vi "Shooter Data.vi"(1 "Wheel Speed":T2, 2 "Arm Angle":T1) -> (0 "Shooter Data":T3)   [LabVIEW 2015]
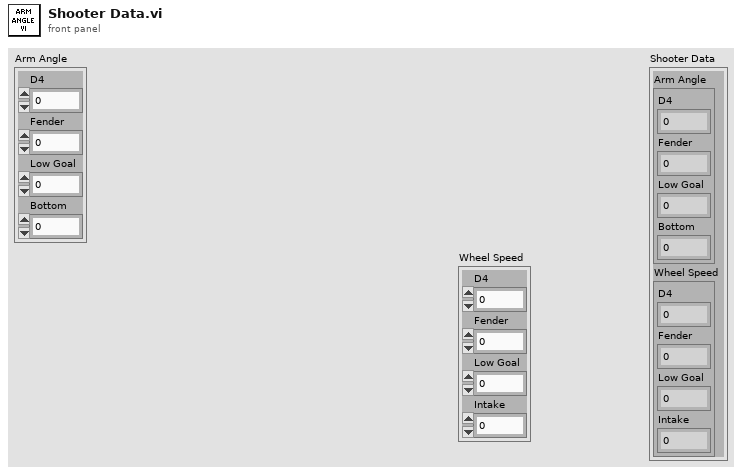
[diagram p1: front panel]
types:
  T1 = cluster{"D4":dbl, "Fender":dbl, "Low Goal":dbl, "Bottom":dbl}
  T2 = cluster{"D4":dbl, "Fender":dbl, "Low Goal":dbl, "Intake":dbl}
  T3 = cluster{"Arm Angle":cluster{"D4":dbl, "Fender":dbl, "Low Goal":dbl, "Bottom":dbl}, "Wheel Speed":cluster{"D4":dbl, "Fender":dbl, "Low Goal":dbl, "Intake":dbl}}
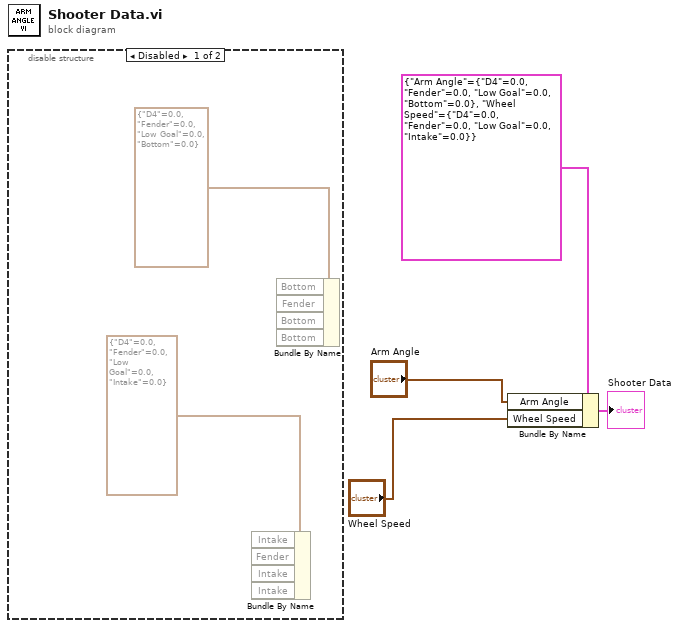
[diagram p0: block diagram]
diagram:
  n1 = disable-structure shown="Disabled" {
    frame Disabled {
      n2 = Bundle By Name(cluster=T2 {"D4"=0.0, "Fender"=0.0, "Low Goal"=0.0, "Intake"=0.0} ("input cluster")) -> ()  [unwired: 4 in, 1 out]
      n3 = Bundle By Name(cluster=T1 {"D4"=0.0, "Fender"=0.0, "Low Goal"=0.0, "Bottom"=0.0} ("input cluster")) -> ()  [unwired: 4 in, 1 out]
    }
    frame Enabled {
    }
  }
  n4 = Bundle By Name(cluster=T3 {"Arm Angle"={"D4"=0.0, "Fender"=0.0, "Low Goal"=0.0, "Bottom"=0.0}, "Wheel Speed"={"D4"=0.0, "Fender"=0.0, "Low Goal"=0.0, "Intake"=0.0}} ("input cluster"), "Arm Angle"="Arm Angle", "Wheel Speed"="Wheel Speed") -> (→"Shooter Data":T3)
